vi "command engine send commands.vi"(8 "error in (no error)":errorcluster, 9 "State Variables":T1, 10 "Parameters":T4 {"Compiled"."External Channels"."Channels" format="%.0x"; "Compiled"."External Channels"."Triggers" format="%.0x"}, 11 "Global Variables":T15) -> (0 "error out":errorcluster, 1 "State Variables out":T1, 2 "Parameters out":T4 {"Compiled"."External Channels"."Channels" format="%.0x"; "Compiled"."External Channels"."Triggers" format="%.0x"}, 3 "Global Variables out":T15)   [LabVIEW 2015, in "Instrument Addon Engine.lvlib"]
uses:
  Instrument Addon Engine.lvlib
  Types/Engine State Variables.ctl
  <vilib>/NI/NI VeriStand Inline Async API/_VS Inline Async API/Process/Process.lvclass
  Types/TCP Refs.ctl
  <vilib>/NI/STM/Connection Manager/TCP/Advanced/TCP Connection Manager Reference.ctl
  <vilib>/NI/STM/Connection Manager/TCP/Advanced/TCP Connection Manager State Variables.ctl
  <vilib>/NI/STM/TCP/TCP Connection Info.ctl
  <vilib>/NI/STM/SubVIs/MetaDataElement.ctl
  <vilib>/NI/STM/Connection Manager/TCP/TCP Connection Properties.ctl
  <vilib>/NI/AMC/Message Queue.ctl
  <vilib>/NI/AMC/Message.ctl
  <vilib>/NI/Tools/Keyed Array/KeyedArray.ctl
  <vilib>/NI/NI VeriStand Inline Async API/_Data Access Engine/Access Type Classes/Write/Write.lvclass
  <vilib>/NI/NI VeriStand Inline Async API/_Data Access Engine/Access Type Classes/Read/Read.lvclass
  <vilib>/NI/NI VeriStand Inline Async API/_Data Access Engine/Access Type Classes/ReadWrite/ReadWrite.lvclass
  Types/command engine global variables.ctl
  Types/Commands RT Configuration Cluster.ctl
  Protocols.lvlibp/Protocol Parent/Protocol Parent.lvclass
  Shared/Types/Compiled Settings.ctl
  Shared/Types/Command Parameters.ctl
  Shared/Types/Linked Channel Cluster.ctl
  Shared/Types/Response RT Configuration Cluster.ctl
  Shared/Types/Response Parameters.ctl
  Shared/Types/Response Wait Type.ctl
  Shared/Types/Message Parameters.ctl
  Shared/Types/Message Generation Type.ctl
  Shared/Types/External Trigger Refs.ctl
  <vilib>/NI Veristand/Custom Device API/Data Reference.ctl
  Protections.lvlibp/Parent Protection/Protection.lvclass
  Format Numeric to String.vi
  <vilib>/NI/Tools/Keyed Array/Tools_KeyedArray.lvlib
  <vilib>/NI/AMC/AMC.lvlib
  Shared/Instrument Addon Shared.lvlib
  <vilib>/NI VeriStand/Custom Device API/Custom Device API.lvlib
  <vilib>/NI/STM/NI STM.lvlib
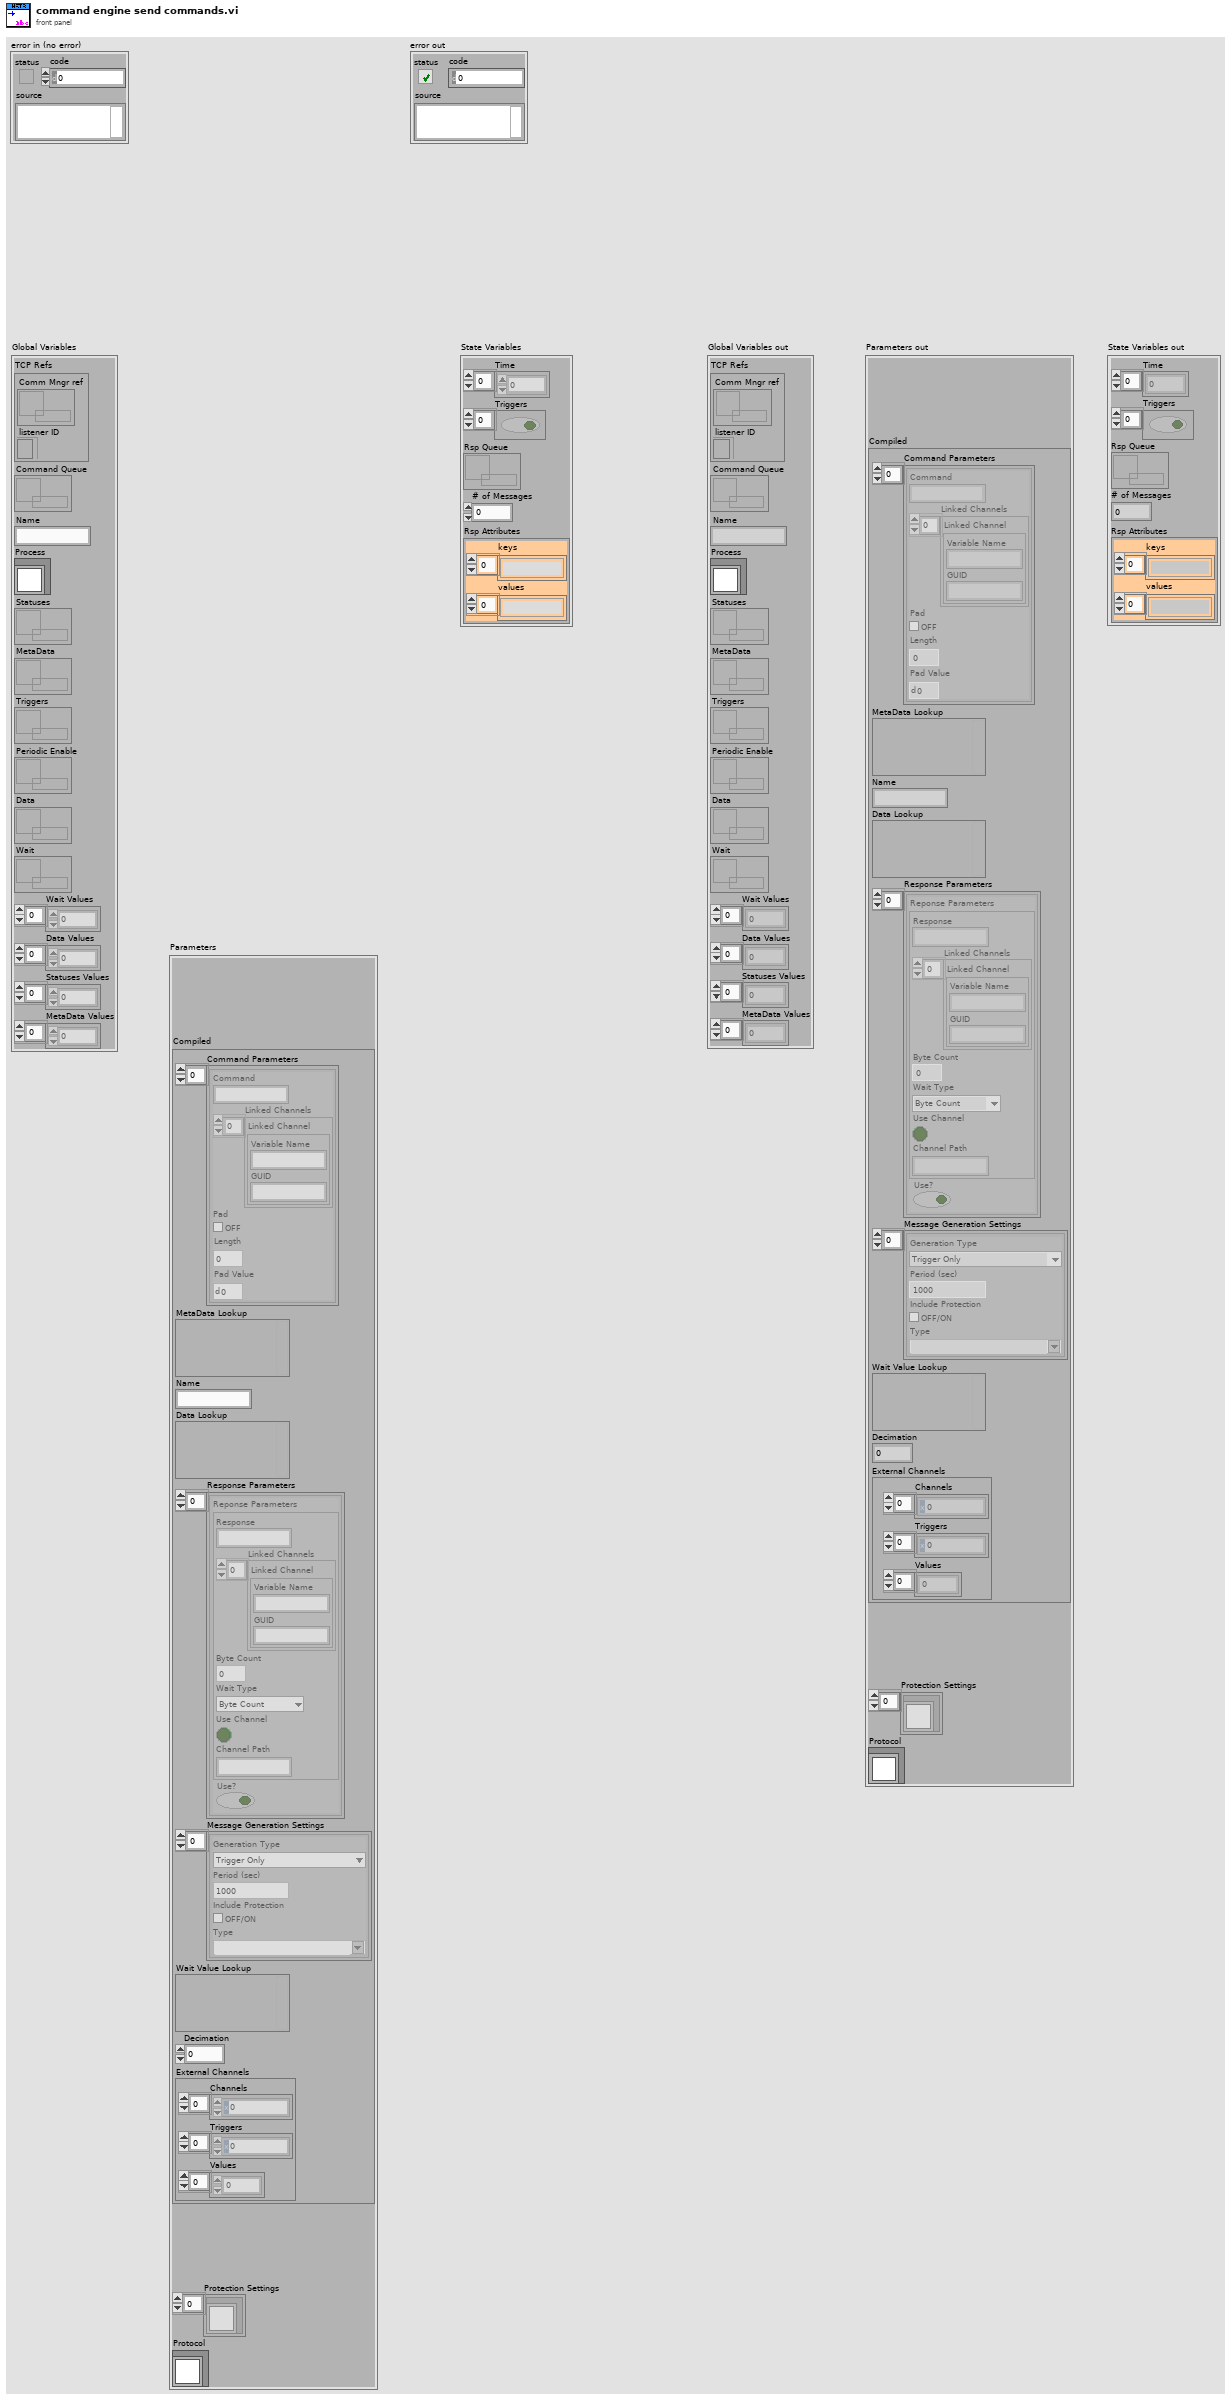
[diagram p1: front panel]
types:
  T1 = typedef "Instrument Addon Engine.lvlib/command engine global variables.ctl" = cluster{"Time":u32[], "Triggers":bool[], "Rsp Queue":T2, "# of Messages":i32, "Rsp Attributes":T3}
  T2 = typedef "AMC.lvlib/Message Queue.ctl" = refnum<queue>
  T3 = typedef "Tools_KeyedArray.lvlib/KeyedArray.ctl" = cluster{"keys":string[], "values":string[]}
  T4 = typedef "Instrument Addon Engine.lvlib/Commands RT Configuration Cluster.ctl" = cluster{"Compiled":T5, "Protection Settings":refnum<class "Protection.lvclass">[], "Protocol":refnum<class "Protocol Parent.lvclass">}
  T5 = typedef "Instrument Addon Shared.lvlib/Compiled Settings.ctl" = cluster{"Command Parameters":T6[], "MetaData Lookup":variant, "Name":string, "Data Lookup":variant, "Response Parameters":T8[], "Message Generation Settings":T11[], "Wait Value Lookup":variant, "Decimation":u32, "External Channels":T13}
  T6 = typedef "Instrument Addon Shared.lvlib/Command Parameters.ctl" = cluster{"Command":string, "Linked Channels":T7[], "Pad":bool, "Length":u32, "Pad Value":u8}
  T7 = typedef "Instrument Addon Shared.lvlib/Linked Channel Cluster.ctl" = cluster{"Variable Name":string, "GUID":string}
  T8 = typedef "Instrument Addon Shared.lvlib/Response RT Configuration Cluster.ctl" = cluster{"Reponse Parameters":T9, "Use?":bool}
  T9 = typedef "Instrument Addon Shared.lvlib/Response Parameters.ctl" = cluster{"Response":string, "Linked Channels":T7[], "Type Value":dbl, "Wait Type":T10, "Use Channel":bool, "Channel Path":string}
  T10 = typedef "Instrument Addon Shared.lvlib/Response Wait Type.ctl" = enum16{"Byte Count", "Wait sec"}
  T11 = typedef "Instrument Addon Shared.lvlib/Message Parameters.ctl" = cluster{"Generation Type":T12, "Period":dbl, "Include Protection":bool, "Type":string}
  T12 = typedef "Instrument Addon Shared.lvlib/Message Generation Type.ctl" = enum16{"Trigger Only", "Periodic & Trigger"}
  T13 = typedef "Instrument Addon Shared.lvlib/External Trigger Refs.ctl" = cluster{"Channels":T14[], "Triggers":T14[], "Values":dbl[]}
  T14 = typedef "Custom Device API.lvlib/Data Reference.ctl" = i32
  T15 = typedef "Instrument Addon Engine.lvlib/Engine State Variables.ctl" = cluster{"TCP Refs":T16, "Command Queue":T2, "Name":string, "Process":refnum<class "Process.lvclass">, "Statuses":refnum<data-value>, "MetaData":refnum<data-value>, "Triggers":refnum<data-value>, "Periodic Enable":refnum<data-value>, "Data":refnum<data-value>, "Wait":refnum<data-value>, "Wait Values":dbl[], "Data Values":dbl[], "Statuses Values":dbl[], "MetaData Values":dbl[]}
  T16 = typedef "Instrument Addon Engine.lvlib/TCP Refs.ctl" = cluster{"Comm Mngr ref":T17, "listener ID":refnum<k5>}
  T17 = typedef "TCP Connection Manager Reference.ctl" = refnum<data-value>
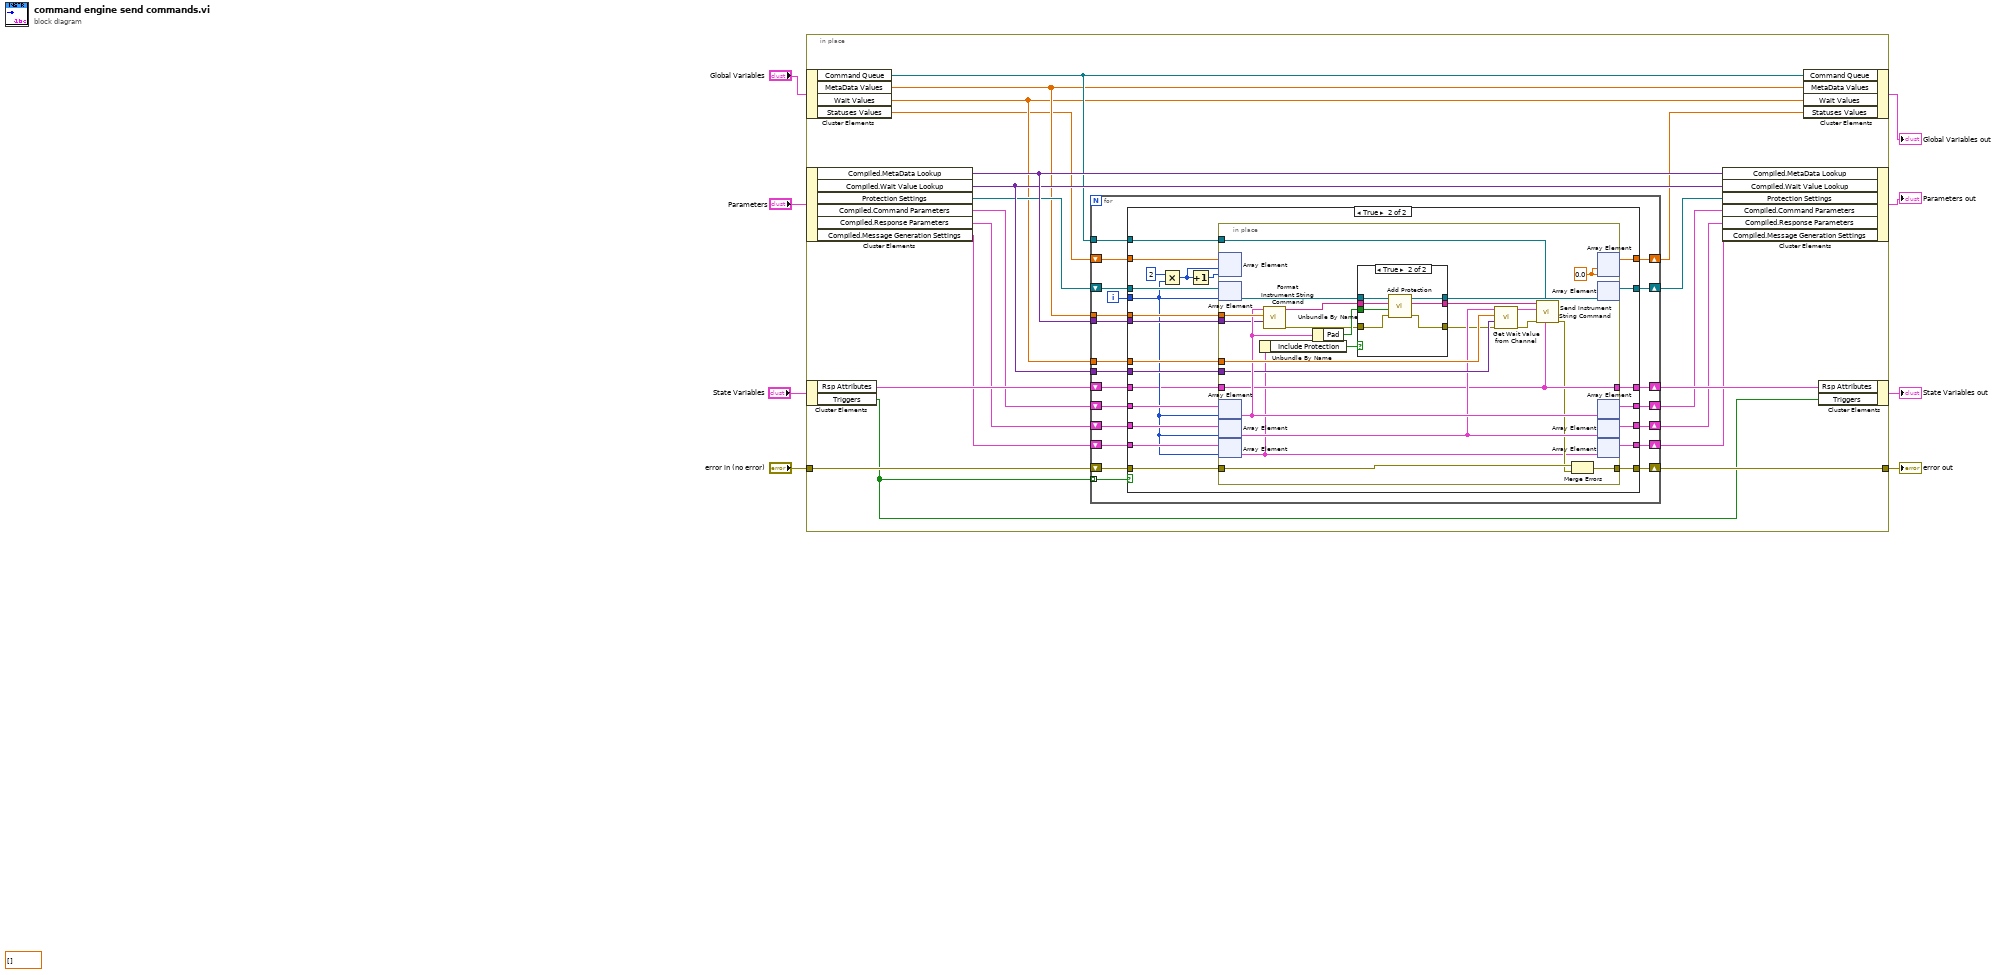
[diagram p0: block diagram]
diagram:
  (unwired) dbl[] []
  n1 = in-place {
    in-place-border: "error in (no error)" -> [w28]
    in-place-border: [w16] -> w4
    n2 = in-place-cluster #1("Global Variables") -> ("Command Queue"=w17:T2, "MetaData Values"=w12:dbl[], "Wait Values"=w11:dbl[], "Statuses Values"=w9:dbl[])
    n3 = in-place-cluster #2("Parameters") -> ("Compiled.MetaData Lookup"=w27:variant, "Compiled.Wait Value Lookup"=w26:variant, "Protection Settings"=w15:refnum<class "Protection.lvclass">[], "Compiled.Command Parameters"=w19:T6[], "Compiled.Response Parameters"=w21:T8[], "Compiled.Message Generation Settings"=w23:T11[])
    n4 = in-place-cluster #3("State Variables") -> ("Rsp Attributes"=w25:T3, "Triggers"=w13:bool[])
    n5 = for {
      shift-right: [w41] -> w10
      shift-left: w9 -> [w42]
      shift-right: [w43] -> w20
      shift-left: w21 -> [w44]
      shift-right: [w39] -> w22
      shift-left: w23 -> [w40]
      shift-right: [w45] -> w14
      shift-left: w15 -> [w46]
      shift-right: [w30] -> w24
      shift-left: w25 -> [w31]
      shift-right: [w37] -> w18
      shift-left: w19 -> [w38]
      tunnel: w26 -> [w47]
      tunnel: w27 -> [w36]
      tunnel: w11 -> [w35]
      tunnel: w12 -> [w34]
      tunnel: w17 -> [w33]
      shift-right: [w48] -> w16
      shift-left: w28 -> [w49]
      tunnel: w13 -> [w29] mode=indexing
      i -> [w32]
      n6 = case shown="True" w29 {
        tunnel: w49 -> [w54 w79]
        tunnel: [w54 w78] -> w48
        tunnel: w47 -> [_ w77]
        tunnel: w46 -> [w55 w76]
        tunnel: [w55 w75] -> w45
        tunnel: w44 -> [w51 w74]
        tunnel: [w51 w73] -> w43
        tunnel: w42 -> [w56 w72]
        tunnel: [w56 w68] -> w41
        tunnel: w40 -> [w50 w67]
        tunnel: [w50 w66] -> w39
        tunnel: w38 -> [w52 w65]
        tunnel: [w52 w64] -> w37
        tunnel: w36 -> [_ w63]
        tunnel: w35 -> [_ w62]
        tunnel: w34 -> [_ w61]
        tunnel: w33 -> [_ w60]
        tunnel: w32 -> [_ w59]
        tunnel: w31 -> [w53 w58]
        tunnel: [w53 w57] -> w30
        frame False {
        }
        frame True {
          n7 = Multiply(x=2, y=w59) -> (x*y=w70:i32)
          n8 = Increment(x=w70) -> (x+1=w69:i32)
          n9 = in-place {
            in-place-border: w79 -> [w102]
            in-place-border: [w101] -> w78
            in-place-border: w61 -> [w94]
            in-place-border: w63 -> [w91]
            in-place-border: w77 -> [w92]
            in-place-border: w62 -> [w95]
            in-place-border: w60 -> [w80]
            in-place-border: w58 -> [w89]
            in-place-border: [w89] -> w57
            w96 = 0.0
            n10 = in-place-array #4(w72, w70, w69) -> ()  [unwired: 2 out]
            n11 = in-place-array #5(w76, w59) -> (w98:refnum<class "Protection.lvclass">)
            n12 = in-place-array #6(w65, w59) -> (w93:T6)
            n13 = in-place-array #7(w74, w59) -> (w90:T8)
            n14 = in-place-array #8(w67, w59) -> (w81:T11)
            n15 = Unbundle By Name(w81) -> ("Include Protection"=w99:bool)
            n16 = call "Format Instrument String Command.vi"("MetaData Lookup in"=w91, "MetaData"=w94, "Command Parameters"=w93) -> ("error out"=w84:errorcluster, "Command"=w85:string)  [unwired: 6 in, 1 out]
            n17 = Unbundle By Name(w93) -> ("Pad"=w100:bool)
            n18 = case shown="True" w99 {
              tunnel: w85 -> [w104 w112]
              tunnel: w84 -> [w105 w111]
              tunnel: [w105 w110] -> w83
              tunnel: [w104 w109] -> w82
              tunnel: w100 -> [_ w108]
              tunnel: w98 -> [w103 w107]
              tunnel: [w103 w106] -> w97
              frame False {
              }
              frame True {
                n19 = call-dynamic "Add Protection.vi"("error in (no error)"=w111, "Pad"=w108, "String in"=w112, "Protection in"=w107) -> ("error out"=w110:errorcluster, "String out"=w109:string, "Protection out"=w106:refnum<class "Protection.lvclass">)  [unwired: 5 in]
              }
            }
            n20 = call "Get Wait Value from Channel.vi"("error in (no error)"=w83, "Wait Value Lookup"=w92, "Wait Values"=w95, "Response"=w90) -> ("error out"=w86:errorcluster, "Response out"=w87:T8)  [unwired: 6 in]
            n21 = call "Send Instrument String Command.vi"("message attributes"=w89, "Command Queue"=w80, "error in (no error)"=w86, "Response Parameters"=w87, "Command"=w82) -> ("error out"=w88:errorcluster)  [unwired: 6 in]
            n22 = Merge Errors(w102, w88) -> (w101:errorcluster)
            n23 = in-place-array #4(w96, w96) -> (w68:dbl[])  [unwired: 2 out]
            n24 = in-place-array #5(w97) -> (w75:refnum<class "Protection.lvclass">[])  [unwired: 1 out]
            n25 = in-place-array #6(w93) -> (w64:T6[])  [unwired: 1 out]
            n26 = in-place-array #7(w90) -> (w73:T8[])  [unwired: 1 out]
            n27 = in-place-array #8(w81) -> (w66:T11[])  [unwired: 1 out]
          }
        }
      }
    }
    n28 = in-place-cluster #2("Compiled.MetaData Lookup"=w27, "Compiled.Wait Value Lookup"=w26, "Protection Settings"=w14, "Compiled.Command Parameters"=w18, "Compiled.Response Parameters"=w20, "Compiled.Message Generation Settings"=w22) -> (→"Parameters out":T4)
    n29 = in-place-cluster #1("Command Queue"=w17, "MetaData Values"=w12, "Wait Values"=w11, "Statuses Values"=w10) -> (→"Global Variables out":T15)
    n30 = in-place-cluster #3("Rsp Attributes"=w24, "Triggers"=w13) -> (→"State Variables out":T1)
  }
  "error out" <- w4
